vi "ADC GUI Disable types.vi"(5 "Tab ref":refnum<vi>, 7 "Enum ref":refnum<vi>, 8 "error in (no error)":errorcluster) -> (0 "error out":errorcluster)   [LabVIEW 2013]
doc: "Disable digitizer types according conditional symbols w_niscope and w_visa."
uses:
  ADC Type.ctl
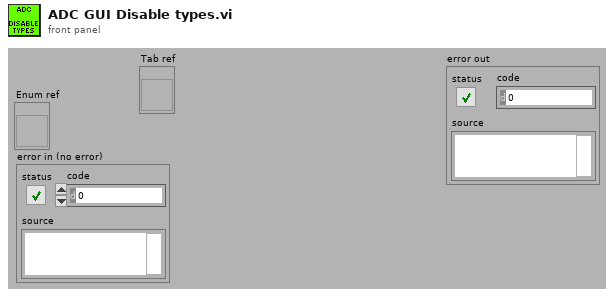
[diagram p1: front panel]
types:
  T1 = typedef "ADC Type.ctl" = enum16{"niScope", "3458A", "DirectSound DLL", "dummy", "QuADC"}
  T2 = enum32{"Page Enabled", "Page Disabled", "Page Disabled & Grayed"}
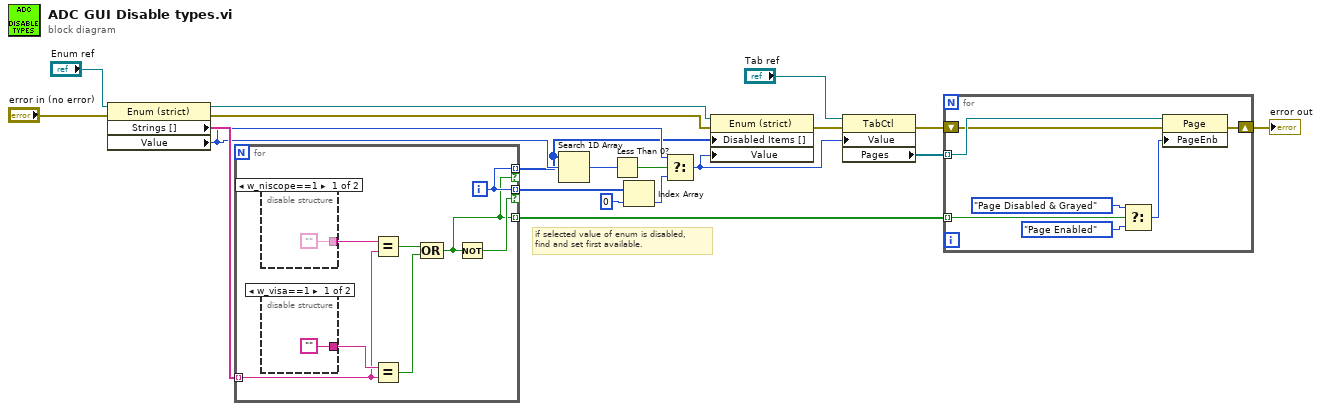
[diagram p0: block diagram]
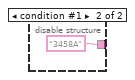
[diagram p2: hidden frame]
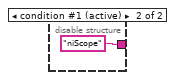
[diagram p3: hidden frame]
diagram:
  # "if selected value of enum is disabled,\nfind and set first available."
  n1 = property class="Enum (strict)"(reference="Enum ref", error in="error in (no error)") -> (reference out=w17:refnum<vi>, error out=w16:errorcluster, "Strings []"=w18:string[], "Value"=w12:T1)
  n2 = for {
    tunnel: w18 -> [w25] mode=indexing
    tunnel: [w21] -> w8 mode=indexing if=w20
    tunnel: [w21] -> w11 mode=indexing if=w22
    tunnel: [w20] -> w5 mode=indexing
    i -> [w21]
    n3 = disable-structure shown="w_niscope==1" {
      disable-tunnel: ["" "niScope"] -> w27
      frame condition #0 {
      }
      frame condition #1 (active) {
      }
    }
    n4 = disable-structure shown="w_visa==1" {
      disable-tunnel: ["" "3458A"] -> w26
      frame condition #0 (active) {
      }
      frame condition #1 {
      }
    }
    n5 = Equal?(x=w27, y=w25) -> (x = y?=w23:bool)
    n6 = Equal?(x=w26, y=w25) -> (x = y?=w24:bool)
    n7 = Compound Arithmetic op=OR(w23, w24) -> (w20:bool)
    n8 = Not(x=w20) -> (.not. x?=w22:bool)
  }
  n9 = Search 1D Array(1D array=w8, element=w12) -> (index of element=w14:i32)  [unwired: 1 in]
  n10 = Less Than 0?(x=w14) -> (x < 0?=w13:bool)
  n11 = Index Array(array=w11, index=u16 0) -> (element=w9:i32)
  n12 = Select(t=w12, s=w13, f=w9) -> (s? t:f=w7:i32)
  n13 = property class="Enum (strict)"(reference=w17, error in=w16, "Disabled Items []"=w8, "Value"=w7) -> (error out=w4:errorcluster)  [unwired: 1 out]
  n14 = property class="TabCtl"(reference="Tab ref", error in=w4, "Value"=w7) -> (error out=w3:errorcluster, "Pages"=w6:refnum<vi>[])  [unwired: 1 out]
  n15 = for {
    tunnel: w6 -> [w38] mode=indexing
    tunnel: w5 -> [w34] mode=indexing
    shift-right: [w32] -> w2
    shift-left: w3 -> [w33]
    n16 = Select(t=T2."Page Disabled & Grayed" ("Page Enabled State"), s=w34, f=T2."Page Enabled" ("Page Enabled State")) -> (s? t:f=w35:T2)
    n17 = property class="Page"(reference=w38, error in=w33, "PageEnb"=w35) -> (error out=w32:errorcluster)  [unwired: 1 out]
  }
  "error out" <- w2
